vi "RSZVB Set UI Data.vi"(8 "error in (no error)":errorcluster {"code" format="%.0x"}, 9 "Data (0)":i32, 10 "Port (A)":i32(ring) items=["A", "B", "C", "D", "E", "F"], 11 "VISA session":refnum<visa-resource-name>) -> (0 "error out":errorcluster {"code" format="%.0x"}, 3 "dup VISA session":refnum<visa-resource-name>)   [LabVIEW 2011]
doc: "This VI write data to ports A, B, C, D, E, F. To write data to a port, the port must be configured as an output port. The port lines have negative logic: A \"0\" at a pin corresponds to a high signal, a \"1\" to a low signal.\n\nRemote-control command(s):\nCONTrol:HANDler:A[:DATA] <decimal>\nCONTrol:HANDler:B[:DATA] <decimal>\nCONTrol:HANDler:C[:DATA] <decimal>\nCONTrol:HANDler:D[:DATA] <decimal>\nCONTrol:HANDler:E[:DATA] <decimal>\nCONTrol:HANDler:F[:DATA] <decimal>"
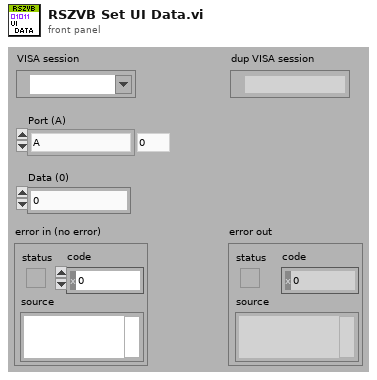
[diagram p1: front panel]
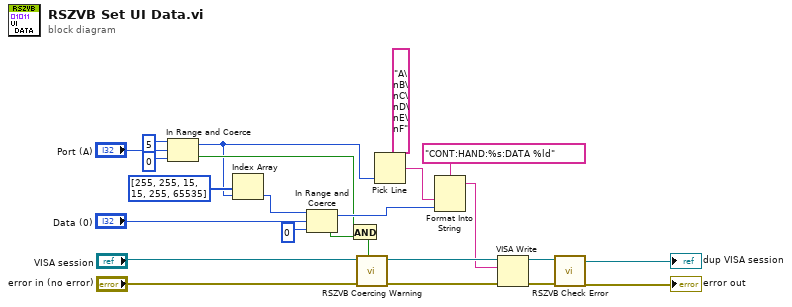
[diagram p0: block diagram]
diagram:
  n1 = In Range and Coerce(upper limit=5, x="Port (A)", lower limit=0) -> (coerced(x)=w2:i32, In Range?=w12:bool)
  n2 = Index Array(array=i32[] [255, 255, 15, 15, 255, 65535], index=w2) -> (element=w1:i32)
  n3 = In Range and Coerce(upper limit=w1, x="Data (0)", lower limit=0) -> (coerced(x)=w13:i32, In Range?=w11:bool)
  n4 = And(x=w12, y=w11) -> (x .and. y?=w10:bool)
  n5 = call "RSZVB Coercing Warning.vi"("In Range?"=w10, "error in (no error)"="error in (no error)", "VISA session"="VISA session") -> ("error out"=w21:errorcluster, "dup VISA session"=w22:refnum<visa-resource-name>)  [unwired: 7 in]
  n6 = Pick Line(multi-line string="A\nB\nC\nD\nE\nF", line index=w2) -> (output string=w14:string)  [unwired: 1 in]
  n7 = Format Into String(format string="CONT:HAND:%s:DATA %ld", w14, w13) -> (resulting string=w18:string)  [unwired: 2 in, 1 out]
  n8 = VISA Write(VISA resource name=w22, write buffer=w18, error in (no error)=w21) -> (VISA resource name out=w19:refnum<visa-resource-name>, error out=w20:errorcluster)  [unwired: 1 out]
  n9 = call "RSZVB Check Error.vi"("error in (no error)"=w20, "VISA session"=w19) -> ("error out"=→"error out":errorcluster, "dup VISA session"=→"dup VISA session":refnum<visa-resource-name>)  [unwired: 8 in]
